vi "StartAsGRPC.vi"(8 "error in":errorcluster, 11 "Service Details":T1) -> (0 "error out":errorcluster, 3 "MicronClient out":refnum<class "MicronClient.lvclass">)   [LabVIEW 2019, in "MicronGRPCClient.lvclass"]
uses:
  MicronGRPCClient.lvclass
  Base/Client/MicronClient.lvclass
  Base/Client/Typedefs/Service Details.ctl
  D:/GitHub/KarthikAbiram/Micron/Source/Base/Client/MicronClient.lvclass
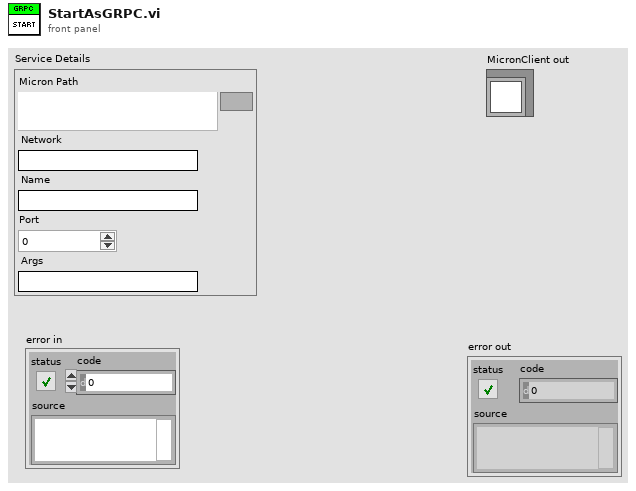
[diagram p1: front panel]
types:
  T1 = typedef "MicronClient.lvclass/Service Details.ctl" = cluster{"Micron Path":path, "Network":string, "Name":string, "Port":i32, "Args":string}
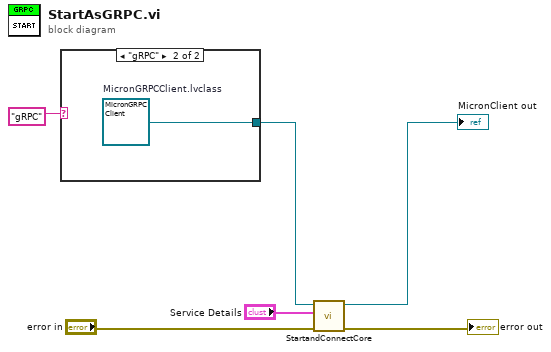
[diagram p0: block diagram]
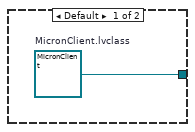
[diagram p2: hidden frame]
diagram:
  n1 = case shown="\"gRPC\"" "gRPC" {
    tunnel: [w7 w8] -> w4
    frame Default {
      w7 = refnum<class "MicronClient.lvclass"> refnum  # MicronClient.lvclass
    }
    frame "gRPC" {
      w8 = refnum<class "MicronGRPCClient.lvclass"> refnum  # MicronGRPCClient.lvclass
    }
  }
  n2 = call-dynamic "StartandConnectCore.vi"("error in (no error)"="error in", "Service Details"="Service Details", "MicronClient in"=w4) -> ("error out"=→"error out":errorcluster, "MicronClient out"=→"MicronClient out":refnum<class "MicronClient.lvclass">)  [unwired: 7 in]
